vi "Method_Const.vi"(4 "Value":u64, 5 "Value A":refnum<class "Abs_U64 Integer.lvclass">) -> (1 "Result":refnum<class "Abs_Boolean.lvclass">)   [LabVIEW 2021, in "Greater Equal_U64.lvclass"]
uses:
  Greater Equal_U64.lvclass
  Abs_Types/U64 Integer/Abs_U64 Integer.lvclass
  Abs_Types/Boolean/Abs_Boolean.lvclass
  C:/TSA/LV_Abstract/Source/Functions/Support/Compare/Two Term/U64/AbsComp_Two Term_U64.lvclass
  C:/Program Files (x86)/National Instruments/LabVIEW 2021/vi.lib/TSA/Abstract Data Classes/Abs_Types/Boolean/Abs_Boolean.lvclass
  Support/Compare/Two Term/U64/AbsComp_Two Term_U64.lvclass/AbsComp_Two Term_U64.ctl
  Support/Compare/Two Term/U64/Properties/Write Numeric A.vi
  Support/Compare/Two Term/U64/Properties/Write Numeric B.vi
  Constants/Support/U64/Const_U64.lvclass
  C:/Program Files (x86)/National Instruments/LabVIEW 2021/vi.lib/TSA/Abstract Data Classes/Abs_Types/Numeric/Abs_Numeric.lvclass
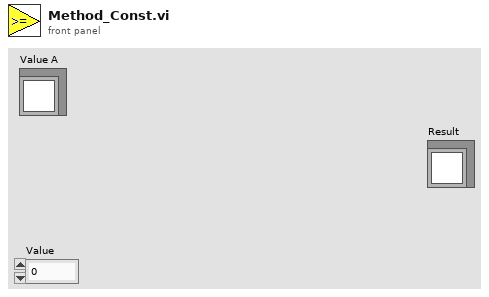
[diagram p1: front panel]
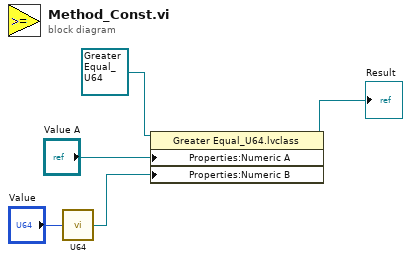
[diagram p0: block diagram]
diagram:
  n1 = call "U64.vi"("Value"="Value") -> ("Constant"=w2:refnum<class "Const_U64.lvclass">)  [unwired: 4 in]
  n2 = property class="Greater Equal_U64.lvclass"(reference=refnum<class "Greater Equal_U64.lvclass"> refnum ("Greater 0_U64.lvclass"), "Properties:Numeric A"="Value A", "Properties:Numeric B"=w2) -> (reference out=→"Result":refnum<class "Greater Equal_U64.lvclass">)  [unwired: 1 in, 1 out]
